vi "EncoderMove.vi"(10 "desiredLeft":dbl, 11 "desiredRight":dbl) -> (0 "desiredLeft(in)":dbl, 1 "encoderLeft(in)":dbl, 2 "desiredRight(in)":dbl, 3 "encoderRight(in)":dbl)   [LabVIEW 2014]
uses:
  <vilib>/Rock Robotics/WPI/RobotDrive/WPI_RobotDriveGetSetRefNum.vi
  Robot Global Data.vi
panel:
  in  "right":dbl
  in  "left":dbl
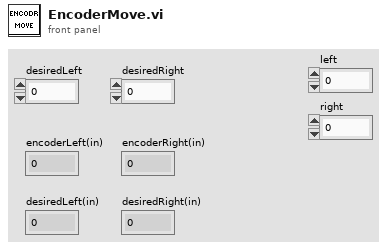
[diagram p1: front panel]
types:
  T1 = typedef "WPI_RobotDriveDevRef.ctl" = cluster{"DevStatus":errorcluster, "Motors[]":T2[], "Square Inputs":bool, "Max Output":dbl}
  T2 = typedef "WPI_MotorControlDeviceRef.ctl" = cluster{"DeviceStatus":errorcluster, "Type":T3, "PWM":cluster{"Controller":T4, "PWM Channel":T5, "DeadBand":T6}, "CAN":cluster{"Device Number":u8, "Control Mode":T7, "Semaphore":T8, "Max Vout":dbl, "TalonSRX Control Mode":T9}, "Invert":bool, "TransformRef":T10, "InvTransformRef":T10}
  T3 = typedef "WPI_MotorControlType.ctl" = enum16{"PWM", "CAN", "CANTalonSRX"}
  T4 = typedef "FPGA_TypedefDigitalModule.ctl" = enum16{"Controller 1"}
  T5 = typedef "FPGA_DIOPWMChannel.ctl" = enum8{"PWM 0", "PWM 1", "PWM 2", "PWM 3", "PWM 4", "PWM 5", "PWM 6", "PWM 7", "PWM 8", "PWM 9", "PWM MXP 0", "PWM MXP 1", "PWM MXP 2", "PWM MXP 3", "PWM MXP 4", "PWM MXP 5", "PWM MXP 6", "PWM MXP 7", "PWM MXP 8", "PWM MXP 9", "Invalid"}
  T6 = typedef "WPI_PWMDeadband.ctl" = cluster{"Name":string, "maxPositivePwm":i32, "minPositivePwm":i32, "centerPwm":i32, "maxNegativePwm":i32, "minNegativePwm":i32, "angularRange":u16}
  T7 = typedef "WPI_CANJaguar_ControlMode.ctl" = enum8{"Percent VBus", "Current", "Speed", "Position", "Voltage"}
  T8 = typedef "Semaphore RefNum" = refnum<k1>
  T9 = typedef "WPI_CANTalonSRX_APIControlMode.ctl" = enum8{"Percent VBus", "Speed", "Position", "Slave", "Unchanged / Invalid"}
  T10 = typedef "WPI_PWMTransform_ConPane.ctl" = refnum<vi>
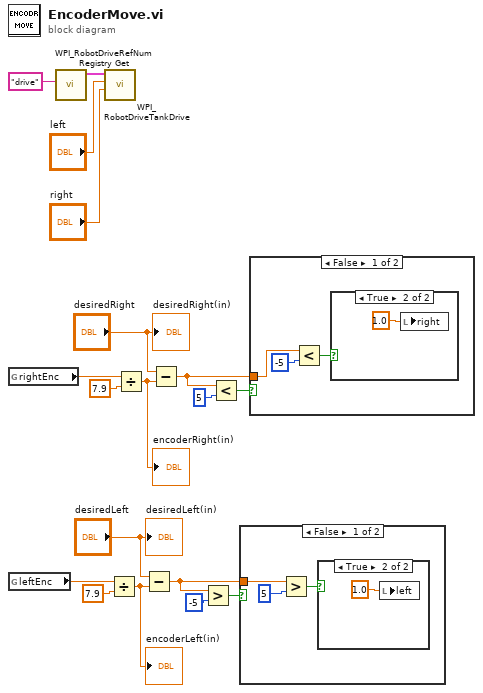
[diagram p0: block diagram]
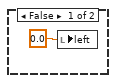
[diagram p2: hidden frame]
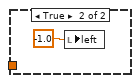
[diagram p3: hidden frame]
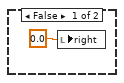
[diagram p4: hidden frame]
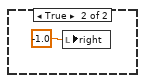
[diagram p5: hidden frame]
diagram:
  n1 = global read "Robot Global Data.vi" "rightEnc"() -> (w16:dbl)
  n2 = global read "Robot Global Data.vi" "leftEnc"() -> (w9:dbl)
  n3 = call <vilib>:"WPI_RobotDriveRefNum Registry Get.vi"("refnum name"="drive") -> ("RobotDriveDevRef"=w4:T1)  [unwired: 9 in, 1 out]
  n4 = call <vilib>:"WPI_RobotDriveTankDrive.vi"("Right axis value"="right", "Left axis value"="left", "RobotDriveDevRef"=w4) -> ()  [unwired: 6 in, 3 out]
  n5 = Divide(x=w9, y=7.9) -> (x/y=w6:dbl)
  "encoderLeft(in)" <- w6
  n6 = Divide(x=w16, y=7.9) -> (x/y=w13:dbl)
  "encoderRight(in)" <- w13
  n7 = Subtract(x="desiredLeft", y=w6) -> (x-y=w5:dbl)
  n8 = Subtract(x="desiredRight", y=w13) -> (x-y=w12:dbl)
  n9 = Greater?(x=w5, y=-5) -> (0:w10:bool)
  n10 = Less?(x=w12, y=5) -> (x < y?=w17:bool)
  n11 = case shown="False" w10 {
    tunnel: w5 -> [w19 _]
    frame False {
      n12 = Greater?(x=w19, y=5) -> (0:w20:bool)
      n13 = case shown="True" w20 {
        frame False {
          n14 = local write "left"(0.0 ("Left axis value")) -> ()
        }
        frame True {
          n15 = local write "left"(1.0 ("Left axis value")) -> ()
        }
      }
    }
    frame True {
      n16 = local write "left"(-1.0 ("Left axis value")) -> ()
    }
  }
  n17 = case shown="False" w17 {
    tunnel: w12 -> [w25 _]
    frame False {
      n18 = Less?(x=w25, y=-5) -> (x < y?=w26:bool)
      n19 = case shown="True" w26 {
        frame False {
          n20 = local write "right"(0.0 ("Left axis value")) -> ()
        }
        frame True {
          n21 = local write "right"(1.0 ("Left axis value")) -> ()
        }
      }
    }
    frame True {
      n22 = local write "right"(-1.0 ("Left axis value")) -> ()
    }
  }
  "desiredRight(in)" <- "desiredRight"
  "desiredLeft(in)" <- "desiredLeft"
